vi "Write Camera Settings to Report File.vi"(8 "error in (no error)":errorcluster, 10 "refnum in":T1, 11 "HIJ IMAQdx Display in":refnum<class "HIJ IMAQdx Display.lvclass">) -> (0 "error out":errorcluster, 2 "refnum out":T1, 3 "HIJ IMAQdx Display out":refnum<class "HIJ IMAQdx Display.lvclass">)   [LabVIEW 2014, in "HIJ IMAQdx Display.lvlib" / "HIJ IMAQdx Display.lvclass"]
uses:
  HIJ IMAQdx Display.lvclass
  <vilib>/Utility/config.llb/Config Data RefNum.ctl
  HIJ IMAQdx Display.lvclass/HIJ IMAQdx Display.ctl
  <vilib>/vision/driver/IMAQdx.llb/IMAQdx Attribute Type.ctl
  <vilib>/Utility/config.llb/Write Key (String).vi
  <vilib>/Utility/config.llb/Write Key (Double).vi
  <vilib>/Utility/config.llb/Write Key (U32).vi
  <vilib>/Utility/config.llb/Write Key (Boolean).vi
  <vilib>/Utility/config.llb/NI_LVConfig.lvlib
  <vilib>/vision/driver/NI_Vision_Acquisition_Software.lvlib
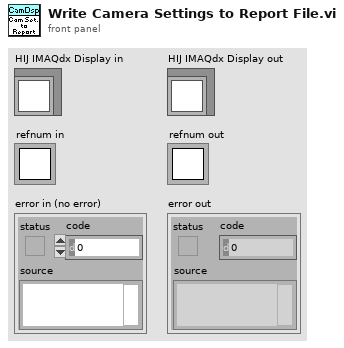
[diagram p1: front panel]
types:
  T1 = typedef "NI_LVConfig.lvlib/Config Data RefNum.ctl" = refnum<k1>
  T2 = typedef "NI_Vision_Acquisition_Software.lvlib/IMAQdx Attribute Type.ctl" = enum32{"U32", "I64", "DBL", "String", "Enum", "Bool", "Command"}
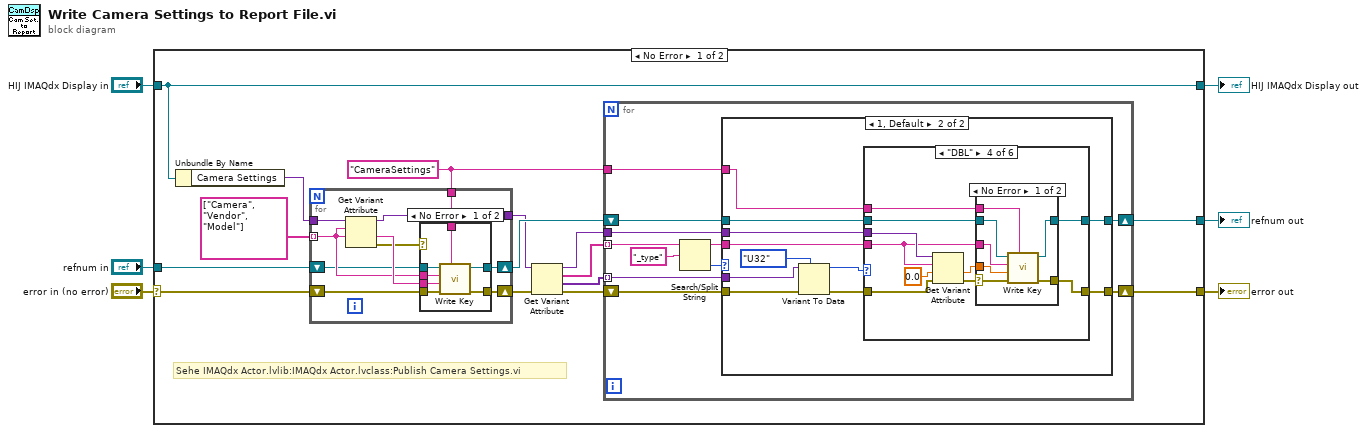
[diagram p0: block diagram]
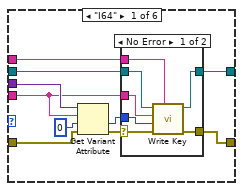
[diagram p4: hidden frame]
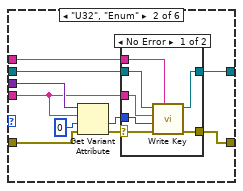
[diagram p6: hidden frame]
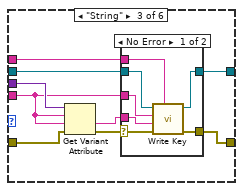
[diagram p8: hidden frame]
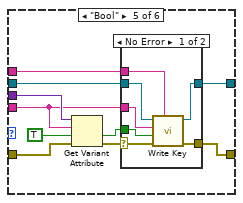
[diagram p11: hidden frame]
diagram:
  n1 = case shown="No Error" "error in (no error)" {
    selector: "error in (no error)" -> [w13 w163]
    tunnel: [w16 w163] -> w5
    tunnel: [w21 w162] -> w3
    tunnel: "HIJ IMAQdx Display in" -> [w21 w162]
    tunnel: "refnum in" -> [w11 w161]
    tunnel: [w17 w161] -> w1
    frame No Error {
      w8 = "CameraSettings"
      # "Sehe IMAQdx Actor.lvlib:IMAQdx Actor.lvclass:Publish Camera Settings.vi"
      n2 = Unbundle By Name(w21) -> ("Camera Settings"=w9:variant)
      n3 = for {
        tunnel: w9 -> [w31]
        tunnel: w8 -> [w29]
        shift-right: [w30] -> w10
        shift-left: w11 -> [w23]
        tunnel: string[] ["Camera", "Vendor", "Model"] -> [w25] mode=indexing
        shift-right: [w27] -> w12
        shift-left: w13 -> [w28]
        tunnel: [w22] -> w7
        n4 = Get Variant Attribute(Variant=w31, name=w25, default value (empty Variant)=w25) -> (duplicate Variant=w22:variant, value=w26:string, error out=w24:errorcluster)  [unwired: 1 in, 1 out]
        n5 = case shown="No Error" w24 {
          tunnel: w23 -> [w38 w40]
          tunnel: [w37 w40] -> w30
          tunnel: w29 -> [w36 _]
          tunnel: w28 -> [w35 w39]
          tunnel: [w34 w39] -> w27
          tunnel: w26 -> [w33 _]
          tunnel: w25 -> [w32 _]
          frame No Error {
            n6 = call-poly <vilib>:"Write Key.vi"("section"=w36, "error in (no error)"=w35, "value"=w33, "key"=w32, "refnum"=w38) -> ("error out"=w34:errorcluster, "refnum out"=w37:T1)  [unwired: 4 in, 1 out]
          }
          frame Error {
          }
        }
      }
      n7 = Get Variant Attribute(Variant=w7, error in=w12) -> (duplicate Variant=w18:variant, names=w20:string[], values=w19:variant[], error out=w15:errorcluster)  [unwired: 2 in]
      n8 = for {
        tunnel: w20 -> [w51] mode=indexing
        tunnel: w19 -> [w47] mode=indexing
        tunnel: w18 -> [w48]
        tunnel: w8 -> [w41]
        shift-right: [w44] -> w17
        shift-left: w10 -> [w45]
        shift-right: [w43] -> w16
        shift-left: w15 -> [w42]
        n9 = Search/Split String(string=w51, search string/char (-)="_type") -> (substring before match=w46:string, offset of match=w49:i32)  [unwired: 1 in, 1 out]
        n10 = case shown="1, Default" w49 {
          tunnel: w48 -> [_ w60]
          tunnel: w47 -> [_ w64]
          tunnel: w46 -> [_ w61]
          tunnel: w45 -> [w53 w59]
          tunnel: [w53 w58] -> w44
          tunnel: [w52 w57] -> w43
          tunnel: w42 -> [w52 w56]
          tunnel: w41 -> [_ w54]
          frame -1 {
          }
          frame 1, Default {
            n11 = Variant To Data(error in=w56, type=IMAQdx_Attribute_Type."U32" ("Attribute Type"), Variant=w64) -> (data=w62:T2, error out=w55:errorcluster)
            n12 = case shown="\"DBL\"" w62 {
              tunnel: w61 -> [w69 w88 w105 w124 w143 _]
              tunnel: w60 -> [w74 w93 w111 w130 w149 _]
              tunnel: w54 -> [w73 w92 w110 w129 w148 _]
              tunnel: w59 -> [w72 w91 w109 w128 w147 w160]
              tunnel: [w67 w86 w106 w125 w144 w160] -> w58
              tunnel: [w66 w85 w104 w122 w141 w159] -> w57
              tunnel: w55 -> [w65 w84 w103 w121 w140 w159]
              frame "I64" {
                n13 = Get Variant Attribute(Variant=w74, name=w69, default value (empty Variant)=i64 0, error in=w65) -> (value=w70:i64, error out=w68:errorcluster)  [unwired: 2 out]
                n14 = case shown="No Error" w68 {
                  selector: w68 -> [w76 w82]
                  tunnel: w73 -> [w81 _]
                  tunnel: w72 -> [w80 w83]
                  tunnel: w70 -> [w79 _]
                  tunnel: w69 -> [w78 _]
                  tunnel: [w77 w83] -> w67
                  tunnel: [w75 w82] -> w66
                  frame No Error {
                    n15 = call-poly <vilib>:"Write Key.vi"("section"=w81, "error in (no error)"=w76, "value"=w79, "key"=w78, "refnum"=w80) -> ("error out"=w75:errorcluster, "refnum out"=w77:T1)  [unwired: 4 in, 1 out]
                  }
                  frame Error {
                  }
                }
              }
              frame "U32", "Enum" {
                n16 = Get Variant Attribute(Variant=w93, name=w88, default value (empty Variant)=u32 0, error in=w84) -> (value=w89:u32, error out=w87:errorcluster)  [unwired: 2 out]
                n17 = case shown="No Error" w87 {
                  selector: w87 -> [w95 w101]
                  tunnel: w92 -> [w100 _]
                  tunnel: w91 -> [w99 w102]
                  tunnel: w89 -> [w98 _]
                  tunnel: w88 -> [w97 _]
                  tunnel: [w96 w102] -> w86
                  tunnel: [w94 w101] -> w85
                  frame No Error {
                    n18 = call-poly <vilib>:"Write Key.vi"("section"=w100, "error in (no error)"=w95, "value"=w98, "key"=w97, "refnum"=w99) -> ("error out"=w94:errorcluster, "refnum out"=w96:T1)  [unwired: 4 in, 1 out]
                  }
                  frame Error {
                  }
                }
              }
              frame "String" {
                n19 = Get Variant Attribute(Variant=w111, name=w105, default value (empty Variant)=w105, error in=w103) -> (value=w108:string, error out=w107:errorcluster)  [unwired: 2 out]
                n20 = case shown="No Error" w107 {
                  selector: w107 -> [w113 w119]
                  tunnel: w110 -> [w118 _]
                  tunnel: w109 -> [w117 w120]
                  tunnel: w108 -> [w116 _]
                  tunnel: w105 -> [w115 _]
                  tunnel: [w114 w120] -> w106
                  tunnel: [w112 w119] -> w104
                  frame No Error {
                    n21 = call-poly <vilib>:"Write Key.vi"("section"=w118, "error in (no error)"=w113, "value"=w116, "key"=w115, "refnum"=w117) -> ("error out"=w112:errorcluster, "refnum out"=w114:T1)  [unwired: 4 in, 1 out]
                  }
                  frame Error {
                  }
                }
              }
              frame "DBL" {
                n22 = Get Variant Attribute(Variant=w130, name=w124, default value (empty Variant)=0.0, error in=w121) -> (value=w127:dbl, error out=w126:errorcluster)  [unwired: 2 out]
                n23 = case shown="No Error" w126 {
                  selector: w126 -> [w132 w138]
                  tunnel: w129 -> [w137 _]
                  tunnel: w128 -> [w136 w139]
                  tunnel: w127 -> [w135 _]
                  tunnel: w124 -> [w134 _]
                  tunnel: [w133 w139] -> w125
                  tunnel: [w131 w138] -> w122
                  frame No Error {
                    n24 = call-poly <vilib>:"Write Key.vi"("section"=w137, "error in (no error)"=w132, "value"=w135, "key"=w134, "refnum"=w136) -> ("error out"=w131:errorcluster, "refnum out"=w133:T1)  [unwired: 4 in, 1 out]
                  }
                  frame Error {
                  }
                }
              }
              frame "Bool" {
                n25 = Get Variant Attribute(Variant=w149, name=w143, default value (empty Variant)=TRUE, error in=w140) -> (value=w146:bool, error out=w145:errorcluster)  [unwired: 2 out]
                n26 = case shown="No Error" w145 {
                  selector: w145 -> [w150 w157]
                  tunnel: w148 -> [w156 _]
                  tunnel: w147 -> [w155 w158]
                  tunnel: w146 -> [w154 _]
                  tunnel: w143 -> [w153 _]
                  tunnel: [w152 w158] -> w144
                  tunnel: [w151 w157] -> w141
                  frame No Error {
                    n27 = call-poly <vilib>:"Write Key.vi"("section"=w156, "error in (no error)"=w150, "value"=w154, "key"=w153, "refnum"=w155) -> ("error out"=w151:errorcluster, "refnum out"=w152:T1)  [unwired: 4 in, 1 out]
                  }
                  frame Error {
                  }
                }
              }
              frame "Command", Default {
              }
            }
          }
        }
      }
    }
    frame Error {
    }
  }
  "error out" <- w5
  "HIJ IMAQdx Display out" <- w3
  "refnum out" <- w1
